vi "Read Current Position.vi"(4 "Units (0: microsteps)":u16(ring) items=["microsteps", "microns", "millimeters", "inches"], 8 "error in (no error)":errorcluster, 9 "Device and Axis":string, 10 "Microstep Size (0)":dbl, 11 "VISA resource name":refnum<visa-resource-name>) -> (0 "error out":errorcluster, 2 "Position":dbl, 3 "VISA resource name out":refnum<visa-resource-name>)   [LabVIEW 2012, in "Zaber A Series.lvlib"]
doc: "Returns the current position. The unit of the value returned depends on the Units input (default is microsteps). For units other than microsteps, a Microstep Size is required for accurate results. You can optionally read from the position of a single device or axis by specifying the Device and Axis input.\n\nThis VI requires that the Initialize VI has been called with the same serial port."
uses:
  <instrlib>/Zaber A Series/Zaber A Series.lvlib
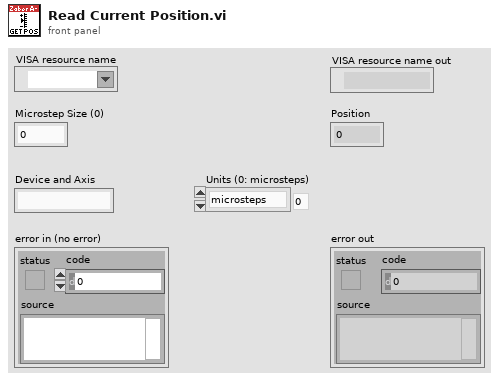
[diagram p1: front panel]
types:
  T1 = cluster{"Device":string, "Axis":string, "Reply Flag":string, "Status":string, "Warning Flags":string, "Data":string}[]
  T2 = cluster{"Device":string, "Axis":string, "Reply Flag":string, "Status":string, "Warning Flags":string, "Data":string}
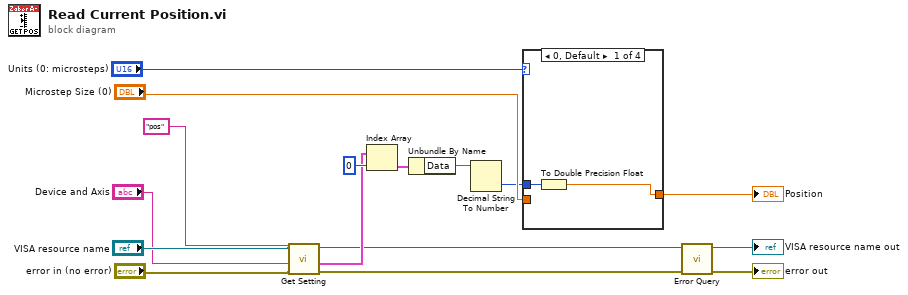
[diagram p0: block diagram]
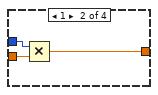
[diagram p2: hidden frame]
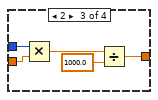
[diagram p3: hidden frame]
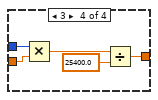
[diagram p4: hidden frame]
diagram:
  n1 = call <instrlib>:"Get Setting.vi"("error in (no error)"="error in (no error)", "Device and Axis"="Device and Axis", "Setting"="pos" ("All Settings (Access Level 2)"), "VISA resource name"="VISA resource name") -> ("error out"=w4:errorcluster, "Response Bundle Array"=w5:T1, "VISA resource name out"=w3:refnum<visa-resource-name>)  [unwired: 3 in, 2 out]
  n2 = Index Array(array=w5, index=0 ("index (row)")) -> (element=w14:T2)
  n3 = Unbundle By Name(w14) -> ("Data"=w13:string)
  n4 = Decimal String To Number(string=w13) -> (number=w12:i32)  [unwired: 2 in, 1 out]
  n5 = case shown="0, Default" "Units (0: microsteps)" {
    tunnel: "Microstep Size (0)" -> [_ w20 w25 w28]
    tunnel: w12 -> [w18 w21 w26 w29]
    tunnel: [w17 w19 w22 w27] -> w11
    frame 0, Default {
      n6 = To Double Precision Float(number=w18) -> (double precision float=w17:dbl)
    }
    frame 1 {
      n7 = Multiply(x=w21, y=w20) -> (x*y=w19:dbl)
    }
    frame 2 {
      n8 = Multiply(x=w26, y=w25) -> (x*y=w23:dbl)
      n9 = Divide(x=w23, y=1000.0) -> (x/y=w22:dbl)
    }
    frame 3 {
      n10 = Multiply(x=w29, y=w28) -> (x*y=w31:dbl)
      n11 = Divide(x=w31, y=25400.0) -> (x/y=w27:dbl)
    }
  }
  "Position" <- w11
  n12 = call <instrlib>:"Error Query.vi"("error in (no error)"=w4, "VISA resource name"=w3) -> ("error out"=→"error out":errorcluster, "VISA resource name out"=→"VISA resource name out":refnum<visa-resource-name>)  [unwired: 6 in, 2 out]
